vi "Client_email_addresses.vi"(0 "Extra People to Email":string[](array[string]), 1 "Client Name Contains":string, 2 "Contact All clients?":bool) -> ()   [LabVIEW 2010]
uses:
  ADAM_Global.vi
  Anemometry/Anemometry Sub Vis/Utilities/Email_transfer_global.vi
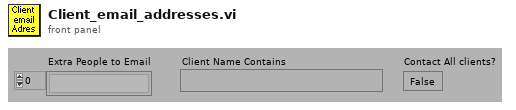
[diagram p1: front panel]
types:
  T1 = typedef "Client_State_Cluster.ctl" = cluster{"Client Name":string, "Traverse level State":T2, "People to Email":string[], "Next Contact Time":dbl}
  T2 = typedef "Traverse_Level_State.ctl" = enum16{"Running", "Complete"}
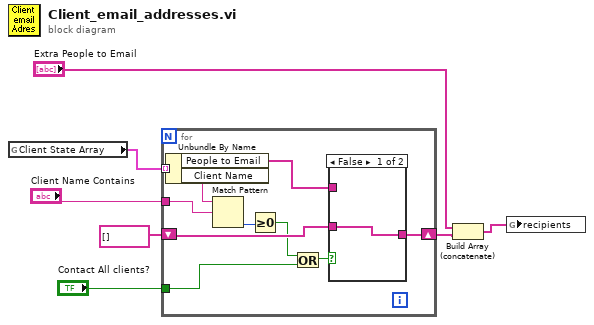
[diagram p0: block diagram]
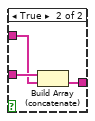
[diagram p2: hidden frame]
diagram:
  n1 = global read "ADAM_Global.vi" "Client State Array"() -> (w1:T1[])
  n2 = for {
    tunnel: w1 -> [w17] mode=indexing
    tunnel: "Client Name Contains" -> [w16]
    shift-right: [w13] -> w5
    shift-left: string[] [] -> [w14]
    tunnel: "Contact All clients?" -> [w8]
    n3 = Unbundle By Name(w17) -> ("People to Email"=w12:string[], "Client Name"=w15:string)
    n4 = Match Pattern(string=w15, regular expression=w16) -> (offset past match=w11:i32)  [unwired: 4 out]
    n5 = Greater Or Equal To 0?(x=w11) -> (x >= 0?=w10:bool)
    n6 = Or(x=w10, y=w8) -> (x .or. y?=w9:bool)
    n7 = case shown="False" w9 {
      tunnel: w14 -> [w18 w21]
      tunnel: [w18 w20] -> w13
      tunnel: w12 -> [_ w19]
      frame False {
      }
      frame True {
        n8 = Build Array (concatenate)(w21, w19) -> (w20:string[])
      }
    }
  }
  n9 = Build Array (concatenate)("Extra People to Email", w5) -> (w7:string[])
  n10 = global write "Email_transfer_global.vi" "recipients"(w7) -> ()
